vi "ttm_status.vi"() -> (2 "statusText":string, 3 "status":i32)   [LabVIEW 2010]
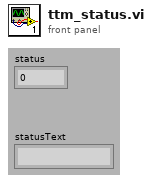
[diagram p1: front panel]
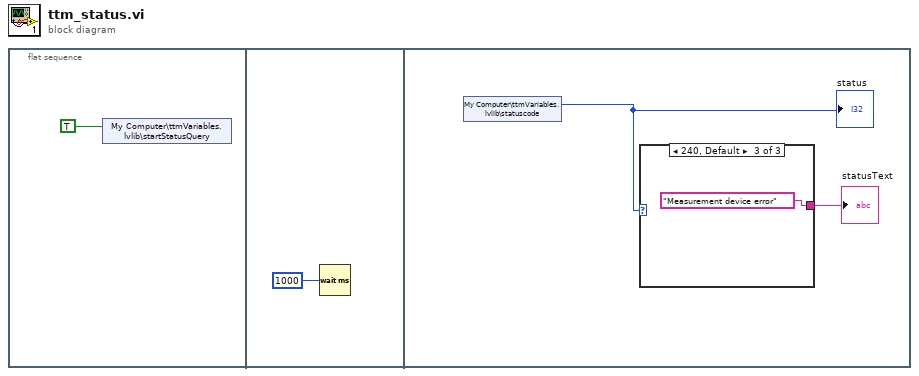
[diagram p0: block diagram]
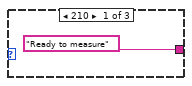
[diagram p2: hidden frame]
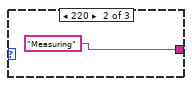
[diagram p3: hidden frame]
diagram:
  n1 = flat-sequence {
    frame #0 {
      n2 = shared-variable "My Computer\\ttmVariables.lvlib\\startStatusQuery"(TRUE ("startStatusQuery")) -> ()  [unwired: 1 in, 1 out]
    }
    frame #1 {
      n3 = Wait (ms)(milliseconds to wait=u32 1000) -> ()  [unwired: 1 out]
    }
    frame #2 {
      n4 = shared-variable "My Computer\\ttmVariables.lvlib\\statuscode"() -> (w3:i32)  [unwired: 1 in, 1 out]
      "status" <- w3
      n5 = case shown="240, Default" w3 {
        tunnel: ["Ready to measure" "Measuring" "Measurement device error"] -> w4
        frame 210 {
        }
        frame 220 {
        }
        frame 240, Default {
        }
      }
      "statusText" <- w4
    }
  }
